vi "StateMachine.vi"() -> ()   [LabVIEW 2011]
doc: "Use this template to build a standard state machine design pattern. Each state executes code and determines which state to transition to. Contrast this design pattern with the User Interface Event Handler pattern, in which code executes in response to user actions. Contrast this design pattern also with the Queued Message Handler pattern, in which each message handling code can queue zero or more new messages."
uses:
  DAQstates.ctl
  <vilib>/DAQmx/read.llb/DAQmx Read (Analog 1D Wfm NChan NSamp).vi
  <vilib>/DAQmx/create/channels.llb/DAQmx Create Channel (AI-Voltage-Basic).vi
  <vilib>/DAQmx/configure/timing.llb/DAQmx Timing (Sample Clock).vi
  <vilib>/DAQmx/miscellaneous.llb/DAQmx Fill In Error Info.vi
  <vilib>/Utility/file.llb/Write To Spreadsheet File (DBL).vi
panel:
  out "Waveform Graph":waveform(dbl)[](graph)
  out "Next State":T1
  in  "Stop":bool
  in  "Save Data":bool
  in  "Take Data":bool
  in  "Channel 2 to read from":tag
  in  "samples per channel":i32=1000
  in  "Rate(Hz)":dbl=1000.0 format="%0.2f"
  in  "Channel 1 to read from":tag
  out "error out":errorcluster
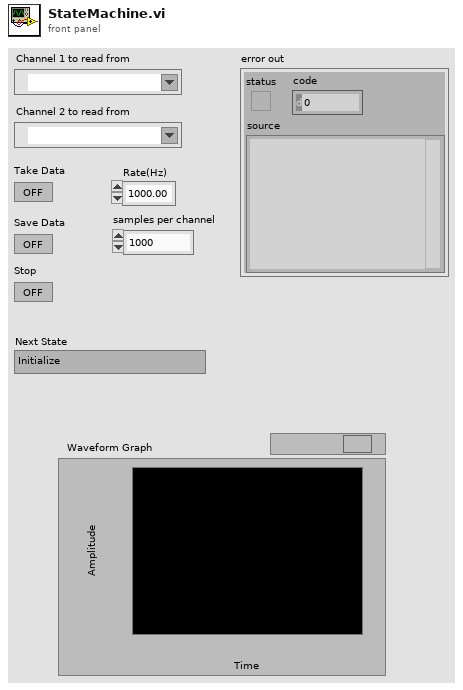
[diagram p1: front panel]
types:
  T1 = typedef "DAQstates.ctl" = enum16{"Initialize", "Wait", "Stop", "Take Data", "Save Data", ""}
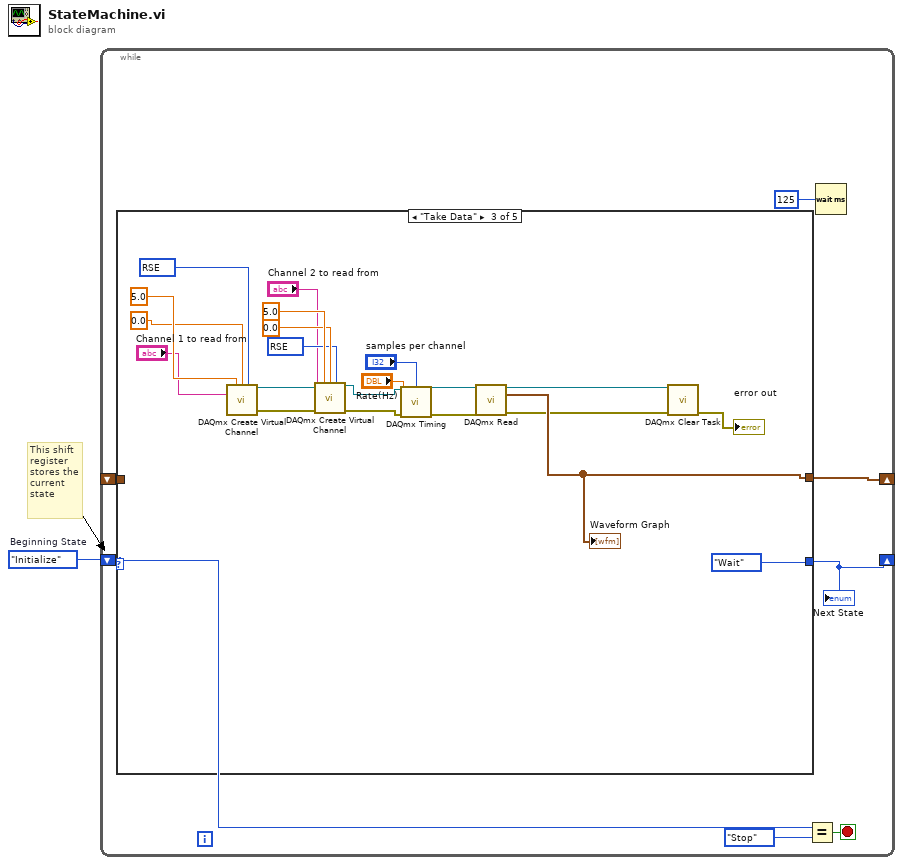
[diagram p0: block diagram]
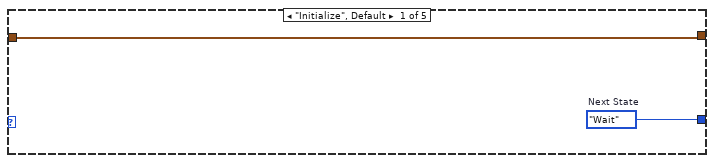
[diagram p2: hidden frame]
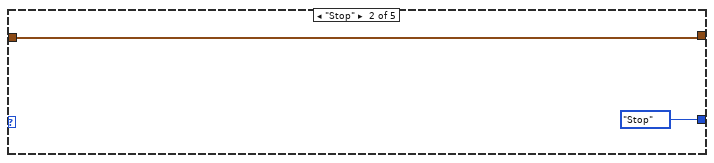
[diagram p3: hidden frame]
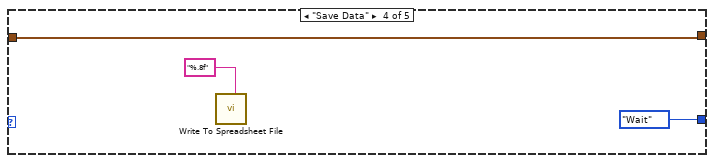
[diagram p4: hidden frame]
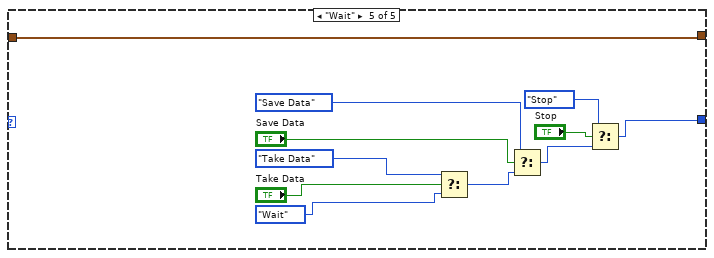
[diagram p5: hidden frame]
diagram:
  w1 = DAQstates."Initialize"  # Beginning State
  # "This shift\nregister\nstores the\ncurrent\nstate"
  n1 = while {
    shift-right: [w5] -> _
    shift-left: w1 -> [w6]
    shift-right: [w2] -> _
    shift-left: _ -> [w3]
    stop <- w8 stop-if-true
    n2 = case shown="\"Take Data\"" w6 {
      tunnel: [w10 DAQstates."Stop" ("Next State") DAQstates."Wait" ("Next State") DAQstates."Wait" ("Next State") w37] -> w5
      tunnel: [w9 w11 w20 w35 w47] -> w2
      tunnel: w3 -> [w9 w11 _ w35 w47]
      frame "Initialize", Default {
        w10 = DAQstates."Wait"  # Next State
      }
      frame "Stop" {
      }
      frame "Take Data" {
        w22 = 10083 items=["default"=-1, "RSE"=10083, "NRSE"=10078, "Differential"=10106, "Pseudodifferential"=12529] ("input terminal configuration")
        w23 = 10083 items=["default"=-1, "RSE"=10083, "NRSE"=10078, "Differential"=10106, "Pseudodifferential"=12529] ("input terminal configuration")
        n3 = call-poly <vilib>:"DAQmx Create Virtual Channel.vi"("maximum value"=5.0, "minimum value"=0.0, "input terminal configuration"=w22, "physical channels"="Channel 1 to read from") -> ("task out"=w29:refnum<k21>, "error out"=w26:errorcluster)  [unwired: 10 in]
        n4 = call-poly <vilib>:"DAQmx Create Virtual Channel.vi"("task in"=w29, "maximum value"=5.0, "minimum value"=0.0, "input terminal configuration"=w23, "physical channels"="Channel 2 to read from", "error in"=w26) -> ("task out"=w18:refnum<k21>, "error out"=w17:errorcluster)  [unwired: 8 in]
        n5 = call-poly <vilib>:"DAQmx Timing.vi"("task/channels in"=w18, "samples per channel"="samples per channel", "rate"="Rate(Hz)", "error in"=w17) -> ("task out"=w15:refnum<k21>, "error out"=w16:errorcluster)  [unwired: 10 in]
        n6 = call-poly <vilib>:"DAQmx Read.vi"("task/channels in"=w15, "error in"=w16) -> ("task out"=w14:refnum<k21>, "data"=w20:waveform(dbl)[], "error out"=w13:errorcluster)  [unwired: 11 in]
        "Waveform Graph" <- w20
        n7 = call <vilib>:"DAQmx Clear Task.vi"("task in"=w14, "error in"=w13) -> ("error out"=→"error out":errorcluster)  [unwired: 13 in]
      }
      frame "Save Data" {
        n8 = call-poly <vilib>:"Write To Spreadsheet File.vi"("format (%.3f)"="%.8f") -> ()  [unwired: 7 in, 1 out]
      }
      frame "Wait" {
        n9 = Select(t=DAQstates."Take Data" ("Next State"), s="Take Data", f=DAQstates."Wait" ("Next State")) -> (s? t:f=w43:T1)
        n10 = Select(t=DAQstates."Save Data" ("Next State"), s="Save Data", f=w43) -> (s? t:f=w40:T1)
        n11 = Select(t=DAQstates."Stop", s="Stop", f=w40) -> (s? t:f=w37:T1)
      }
    }
    "Next State" <- w5
    n12 = Equal?(x=w6, y=DAQstates."Stop" ("States")) -> (x = y?=w8:bool)
    n13 = Wait (ms)(milliseconds to wait=u32 125) -> ()  [unwired: 1 out]
  }
